vi "CRD HF.vi"() -> (0 "error out":errorcluster)   [LabVIEW 2015]
uses:
  <vilib>/rvi/eio/common/nirviEmuClasses.ctl
  <vilib>/rvi/Emulation/niFpgaGetClockAttributes.vi
  <vilib>/rvi/Emulation/niFpgaSctlEmulationGetInTimedLoop.vi
  <vilib>/rvi/Emulation/niFpgaEmulationReportErrorSimple.vi
  <vilib>/rvi/Emulation/niFpgaEmulationIsFPGAContextNoSignature.vi
  <vilib>/rvi/DataTransferAndStorage/Container/Common/niFpgaContainerGetUniqueNameForEmu.vi
  <vilib>/rvi/Memory/Memory_Emulation/niFpgaMemoryEmulationCacheClearOnFirstRun.vi
  <vilib>/rvi/Memory/Memory_Emulation/nirvimemoryEmulationManagerCache_MakeExclusive.vi
  <vilib>/rvi/Memory/Memory_Emulation/niFpgaMemoryEmulationValidateCache.vi
  <vilib>/rvi/Memory/Memory_Emulation/nirvimemoryEmulationManagerCache_InsertValue.vi
  <vilib>/Utility/error.llb/Clear Errors.vi
  <vilib>/rvi/Memory/Memory_Emulation/nirvimemoryEmulationManagerCache_ReleaseExclusive.vi
  <vilib>/rvi/Memory/Memory_Emulation/nirvimemoryEmulationManagerCache_GetValue.vi
  <vilib>/rvi/Memory/Memory_Emulation/nirvimemoryEmulationManagerCache_SetValue.vi
  <vilib>/rvi/Emulation/niFpgaProcessEmulError.vi
  <vilib>/rvi/FIFO/Fifo_Resource/nirvififoEmulationSetSize.vi
  <vilib>/rvi/FIFO/Fifo_Resource/nirviFifoEmulationQueueMgr.vi
  <instcachedir>/0/nirviFifoEmulationQueueMgr_E5CAEC123FF24DC58D834DCA3CDAA9B5.lvgen/nirviFifoEmulationQueueMgr_E5CAEC123FF24DC58D834DCA3CDAA9B5_001.vi
  <vilib>/rvi/errors/niFpgaSetErrorForExecOnDevCompSimple.vi
  <vilib>/rvi/eio/common/nirviEmuReportErrorAndStop.vi
  <vilib>/rvi/FIFO/Fifo_Resource/nirvififoEmulationCreateLock.vi
  <vilib>/rvi/FIFO/Fifo_Resource/nirvififoEmulationObtainLock.vi
  <vilib>/rvi/FIFO/Fifo_Resource/nirvififoEmulationReleaseLock.vi
  <vilib>/rvi/occurrence/nirviWaitOnOccurrenceBase.vi
  <vilib>/rvi/errors/nirviReportUnexpectedCaseInternalError.vi
  <vilib>/rvi/errors/nirviReportUnexpectedCaseInternalError (U32).vi
  <vilib>/rvi/DataTransferAndStorage/Container/Common/niFpgaContainerExecOnDevCompGetState.vi
  <vilib>/rvi/FIFO/Fifo_Resource/nirvififoEmulationDetermineInputValidOut.vi
  <vilib>/rvi/interface/RandomDataEmulation/niFpgaRandomDataHandleErrors.vi
  <vilib>/rvi/Memory/Memory_Emulation/nirvimemoryFastEmulation.vi
  <vilib>/rvi/Memory/Memory_Emulation/nirvimemoryEmulation.vi
  <vilib>/rvi/Emulation/niFpgaCriticalErrorInLSC.vi
  <vilib>/rvi/eio/common/nirviEmuTemplateMethod_errors.vi
  <vilib>/rvi/DataTransferAndStorage/Container/XNode/niFpgaContainer.xnode
  <vilib>/rvi/DataTransferAndStorage/Register/Emulation/niFpgaRegisterEmulation.vi
  <vilib>/rvi/FIFO/Fifo_Resource/nirvififoEmulationGetNumberOfElementsToRead.vi
  <vilib>/rvi/FIFO/Fifo_Resource/nirvififoEmulationRead.vi
  <vilib>/rvi/FIFO/Fifo_Resource/niFpgaFifoEmulationRefIn.vi
  <vilib>/rvi/interface/RandomDataEmulation/nirviRandomDataFpgaReadWriteTemplate.vi
  <vilib>/eio/EIOGrowableMethodNode/genericMethod/EIOGrowableMethodNode.xnode
  <vilib>/rvi/eio/nirviEIOMethodImplementation/nirviEIOMethodImplementation.xnode
  <vilib>/rvi/eio/nirviErrorMerge/nirviErrorMerge.xnode
  <vilib>/eio/EIONode/EIONode.xnode
  <vilib>/rvi/FIFO/Fifo_Resource/nirvififoEmulationWrite.vi
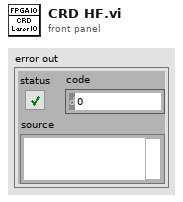
[diagram p1: front panel]
types:
  T1 = typedef "nirviEmuClasses.ctl" = enum16{"IO Read", "IO Write", "Method", "Property Read", "Property Write"}
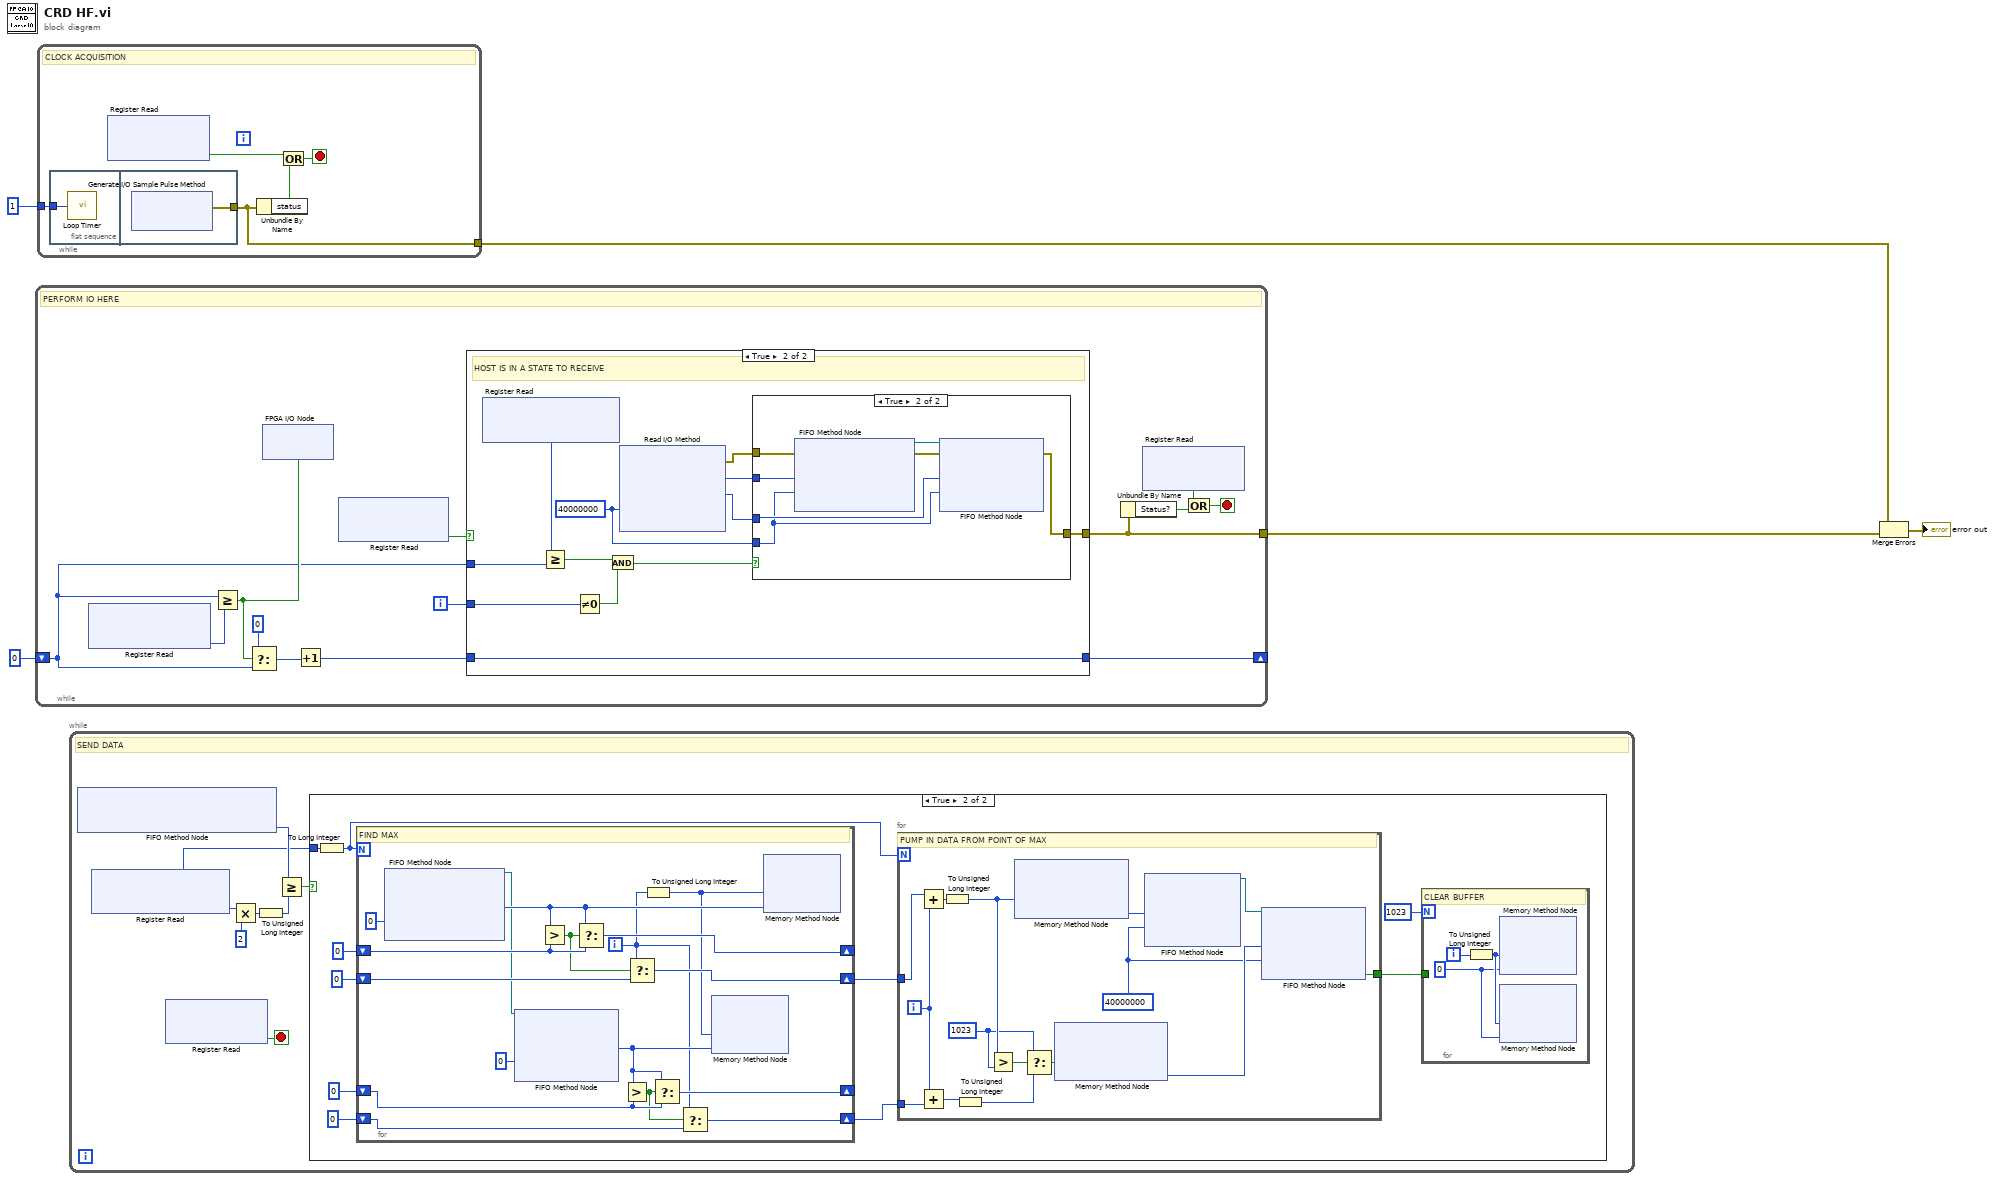
[diagram p0: block diagram]
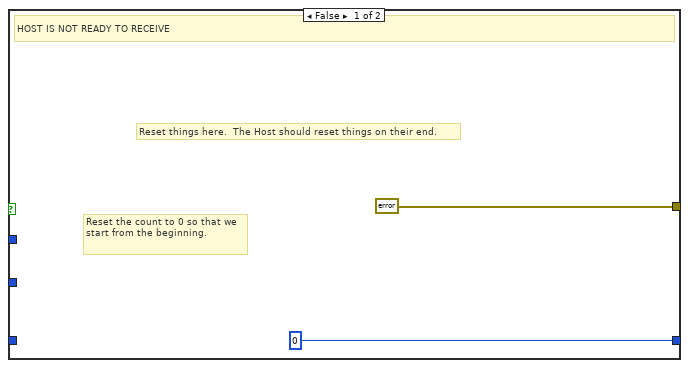
[diagram p3: hidden frame]
diagram:
  n1 = while {
    shift-right: [w11] -> _
    shift-left: u16 0 ("Number of Samples") -> [w12]
    tunnel: [w16] -> w1
    i -> [w7]
    stop <- w10 stop-if-true
    # "PERFORM IO HERE"
    n2 = xnode ("Register Read")() -> ("Data"=w13:u16)  [unwired: 1 in, 1 out]
    n3 = Greater Or Equal?(x=w12, y=w13) -> (x >= y?=w15:bool)
    n4 = Select(t=u16 0 ("Number of Samples"), s=w15, f=w12) -> (s? t:f=w9:u16)
    n5 = xnode "FPGA I/O Node"("CRDS"=w15) -> ()  [unwired: 1 in, 1 out]
    n6 = Increment(x=w9) -> (x+1=w8:u16)
    n7 = xnode ("Register Read")() -> ("Data"=w6:bool)  [unwired: 1 in, 1 out]
    n8 = case shown="True" w6 {
      tunnel: [errorcluster {"Status?"=FALSE, "Code"=0, "Source"=""} ("error out") w26] -> w16
      tunnel: w12 -> [_ w24]
      tunnel: w8 -> [_ w32]
      tunnel: [u16 0 ("Number of Samples") w32] -> w11
      tunnel: w7 -> [_ w27]
      frame False {
        # "Reset things here.  The Host should reset things on their end."
        # "Reset the count to 0 so that we start from the beginning."
        # "HOST IS NOT READY TO RECEIVE"
      }
      frame True {
        w25 = 40000000 ("Timeout")
        # "HOST IS IN A STATE TO RECEIVE"
        n9 = xnode ("Register Read")() -> ("Data"=w23:u16)  [unwired: 1 in, 1 out]
        n10 = Greater Or Equal?(x=w23, y=w24) -> (x >= y?=w22:bool)
        n11 = Not Equal To 0?(x=w27) -> (x != 0?=w29:bool)
        n12 = And(x=w22, y=w29) -> (x .and. y?=w28:bool)
        n13 = xnode "Read I/O Method"("Timeout"=w25) -> ("error out"=w21:errorcluster, "CRD Las Ch 1"=w31:i16, "CRD Las Ch 2"=w30:i16)  [unwired: 3 in, 3 out]
        n14 = case shown="True" w28 {
          tunnel: w31 -> [_ w39]
          tunnel: w30 -> [_ w37]
          tunnel: [_ w35] -> w26
          tunnel: w25 -> [_ w34]
          tunnel: w21 -> [_ w33]
          frame False {
          }
          frame True {
            n15 = xnode ("FIFO Method Node")("Element"=w39, "Timeout"=w34, "error in (no error)"=w33) -> ("error out"=w36:errorcluster, "FIFO Out"=w38:refnum<k21>)  [unwired: 1 in, 1 out]
            n16 = xnode ("FIFO Method Node")("Element"=w37, "Timeout"=w34, "error in (no error)"=w36, "FIFO In"=w38) -> ("error out"=w35:errorcluster)  [unwired: 2 out]
          }
        }
      }
    }
    n17 = Unbundle By Name(w16) -> ("Status?"=w18:bool)
    n18 = xnode ("Register Read")() -> ("Data"=w14:bool)  [unwired: 1 in, 1 out]
    n19 = Compound Arithmetic op=OR(w14, w18) -> (w10:bool)
  }
  n20 = while {
    tunnel: u32 1 ("Sample Period (uSec)") -> [w152]
    tunnel: [w151] -> w5
    stop <- w148 stop-if-true
    # "CLOCK ACQUISITION"
    n21 = flat-sequence {
      tunnel: w152 -> [w153]
      tunnel: [w154] -> w151
      frame #0 {
        n22 = call "Loop Timer"("Count(uSec)"=w153) -> ()  [unwired: 1 out]
      }
      frame #1 {
        n23 = xnode "Generate I/O Sample Pulse Method"() -> ("error out"=w154:errorcluster)  [unwired: 2 in, 1 out]
      }
    }
    n24 = xnode ("Register Read")() -> ("Data"=w150:bool)  [unwired: 1 in, 1 out]
    n25 = Unbundle By Name(w151) -> ("status"=w149:bool)
    n26 = Or(x=w150, y=w149) -> (x .or. y?=w148:bool)
  }
  n27 = while {
    stop <- w201 stop-if-true
    # "SEND DATA"
    n28 = xnode ("FIFO Method Node")() -> ("Number of Elements to Read"=w205:u32)  [unwired: 1 in, 1 out]
    n29 = xnode ("Register Read")() -> ("Data"=w199:u16)  [unwired: 1 in, 1 out]
    n30 = xnode ("Register Read")() -> ("Data"=w201:bool)  [unwired: 1 in, 1 out]
    n31 = Multiply(x=w199, y=u16 2) -> (x*y=w200:u16)
    n32 = To Unsigned Long Integer(number=w200) -> (unsigned 32bit integer=w202:u32)
    n33 = Greater Or Equal?(x=w205, y=w202) -> (x >= y?=w204:bool)
    n34 = case shown="True" w204 {
      tunnel: w199 -> [_ w206]
      frame False {
      }
      frame True {
        n35 = To Long Integer(number=w206) -> (32bit integer=w210:i32)
        n36 = for {
          N: w210 -> [_]
          shift-right: [w247] -> _
          shift-left: i16 0 ("Element") -> [w248]
          shift-right: [w244] -> w213
          shift-left: 0 -> [w245]
          shift-right: [w234] -> w207
          shift-left: 0 -> [w235]
          shift-right: [w239] -> _
          shift-left: i16 0 ("Element") -> [w238]
          i -> [w236]
          # "FIND MAX"
          n37 = xnode ("FIFO Method Node")("Timeout"=0) -> ("Element"=w249:i16, "FIFO Out"=w243:refnum<k21>)  [unwired: 1 in, 1 out]
          n38 = xnode ("FIFO Method Node")("Timeout"=0, "FIFO In"=w243) -> ("Element"=w240:i16)  [unwired: 2 out]
          n39 = Greater?(x=w249, y=w248) -> (0:w246:bool)
          n40 = Select(t=w249, s=w246, f=w248) -> (s? t:f=w247:i16)
          n41 = Greater?(x=w240, y=w238) -> (0:w237:bool)
          n42 = Select(t=w236, s=w246, f=w245) -> (s? t:f=w244:i32)
          n43 = To Unsigned Long Integer(number=w236) -> (unsigned 32bit integer=w241:u32)
          n44 = Select(t=w240, s=w237, f=w238) -> (s? t:f=w239:i16)
          n45 = Select(t=w236, s=w237, f=w235) -> (s? t:f=w234:i32)
          n46 = xnode ("Memory Method Node")("Address"=w241, "Data"=w240) -> ()  [unwired: 1 in, 1 out]
          n47 = xnode ("Memory Method Node")("Address"=w241, "Data"=w249) -> ()  [unwired: 1 in, 1 out]
        }
        n48 = for {
          N: w210 -> [_]
          tunnel: w213 -> [w233]
          tunnel: [w222] -> w211
          tunnel: w207 -> [w228]
          i -> [w229]
          w227 = u32 1023
          w223 = 40000000 ("Timeout")
          # "PUMP IN DATA FROM POINT OF MAX"
          n49 = Add(x=w233, y=w229) -> (x+y=w232:i32)
          n50 = Add(x=w229, y=w228) -> (x+y=w220:i32)
          n51 = To Unsigned Long Integer(number=w232) -> (unsigned 32bit integer=w231:u32)
          n52 = To Unsigned Long Integer(number=w220) -> (unsigned 32bit integer=w219:u32)
          n53 = Greater?(x=w231, y=w227) -> (0:w230:bool)
          n54 = xnode ("Memory Method Node")("Address"=w231) -> ("Data"=w226:i16)  [unwired: 1 in, 1 out]
          n55 = Select(t=w227, s=w230, f=w219) -> (s? t:f=w221:u32)
          n56 = xnode ("Memory Method Node")("Address"=w221) -> ("Data"=w224:i16)  [unwired: 1 in, 1 out]
          n57 = xnode ("FIFO Method Node")("Element"=w226, "Timeout"=w223) -> ("FIFO Out"=w225:refnum<k21>)  [unwired: 1 in, 1 out]
          n58 = xnode ("FIFO Method Node")("Element"=w224, "Timeout"=w223, "FIFO In"=w225) -> ("Timed Out?"=w222:bool)  [unwired: 1 out]
        }
        n59 = for {
          N: 1023 -> [_]
          tunnel: w211 -> [_]
          i -> [w218]
          w216 = i16 0 ("Data")
          # "CLEAR BUFFER"
          n60 = To Unsigned Long Integer(number=w218) -> (unsigned 32bit integer=w217:u32)
          n61 = xnode ("Memory Method Node")("Address"=w217, "Data"=w216) -> ()  [unwired: 1 in, 1 out]
          n62 = xnode ("Memory Method Node")("Address"=w217, "Data"=w216) -> ()  [unwired: 1 in, 1 out]
        }
      }
    }
  }
  n63 = Merge Errors(w5, w1) -> (→"error out":errorcluster)
